vi "expression using methods.vi"() -> ()   [LabVIEW 2022 SP3]
uses:
  <vilib>/express/express arith-compare/Formula/XNode/ExpressFormulaBlockNode.xnode
panel:
  out "Numeric 3":dbl
  out "Numeric 2":dbl
  out "EXPRESS NODE":dbl
  out "FUCTIONS":dbl
  in  "Numeric":dbl
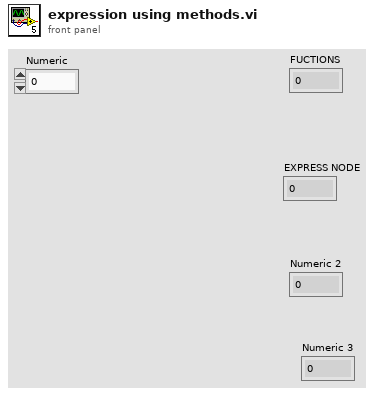
[diagram p1: front panel]
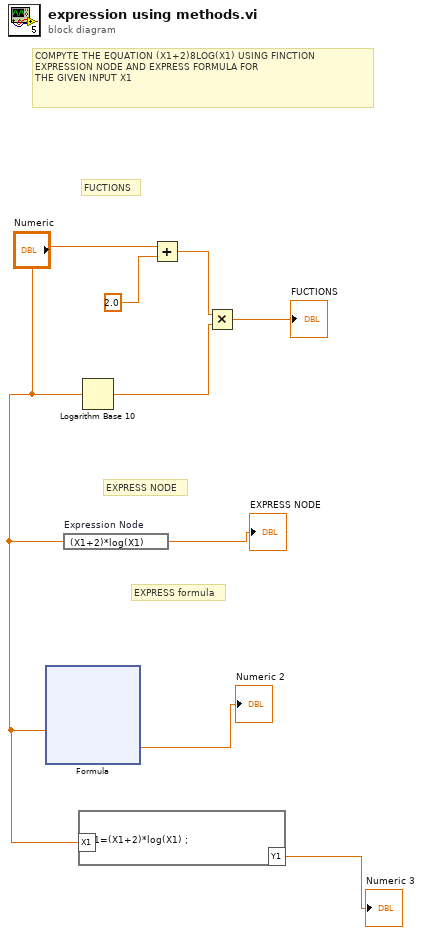
[diagram p0: block diagram]
diagram:
  # "EXPRESS formula"
  # "EXPRESS NODE"
  # "FUCTIONS"
  # "COMPYTE THE EQUATION (X1+2)8LOG(X1) USING FINCTION EXPRESSION NODE AND EXPRESS FORMULA FOR\nTHE GIVEN INPUT X1"
  n1 = xnode "Formula"("X1"="Numeric") -> ("Result"=→"Numeric 2":dbl)  [unwired: 1 in, 1 out]
  n2 = expression code="(X1+2)*log(X1)"("Numeric") -> (→"EXPRESS NODE":dbl)
  n3 = formula code="Y1=(X1+2)*log(X1) ;"("X1"="Numeric") -> ("Y1"=→"Numeric 3":dbl)
  n4 = Logarithm Base 10(1:"Numeric") -> (0:w6:dbl)
  n5 = Add(x="Numeric", y=2.0) -> (x+y=w7:dbl)
  n6 = Multiply(x=w7, y=w6) -> (x*y=→"FUCTIONS":dbl)
